vi "Main.vi"(8 "error in (no error)":errorcluster, 11 "ExampleClassC in":refnum<class "ExampleClassC.lvclass">) -> (0 "error out":errorcluster, 3 "component":refnum<class "ExampleClassC.lvclass">)   [LabVIEW 2012, in "ExampleClassC.lvclass"]
doc: "Main VI of the component. This should contain the GUI of your component and be called when creating an executable."
uses:
  ExampleClassC.lvclass
  <vilib>/Distrio/Murmex/InitialiseMessage/InitialiseMessage.lvclass
  ExampleClassC.lvclass/ExampleClassC.ctl
  <vilib>/Distrio/Murmex/TerminateMessage/TerminateMessage.lvclass
  <vilib>/Distrio/Murmex/ConfigureMessage/ConfigureMessage.lvclass
  <vilib>/Distrio/Murmex/StopMessage/StopMessage.lvclass
  <vilib>/Distrio/Murmex/StartMessage/StartMessage.lvclass
  <vilib>/Distrio/Murmex/Murmex/Set log reference.vi
  <vilib>/Distrio/Murmex/Murmex/Set VI reference.vi
  <vilib>/Distrio/Murmex/Murmex/Set configure at initialise.vi
  <vilib>/Distrio/Murmex/Murmex/Set relay start stop to observers.vi
  <vilib>/Distrio/Murmex/Murmex/Murmex.lvclass
  <vilib>/Distrio/Murmex/Message/Message.lvclass
panel:
  in  "button:configure":bool
  in  "button:start":bool
  in  "image":path
  in  "button:quit":bool
  in  "terminate?":bool
  in  "ID":string
  out "log":string
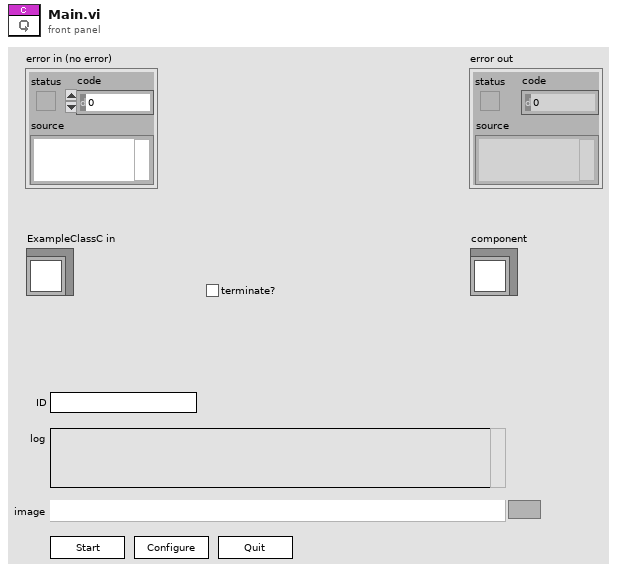
[diagram p1: front panel]
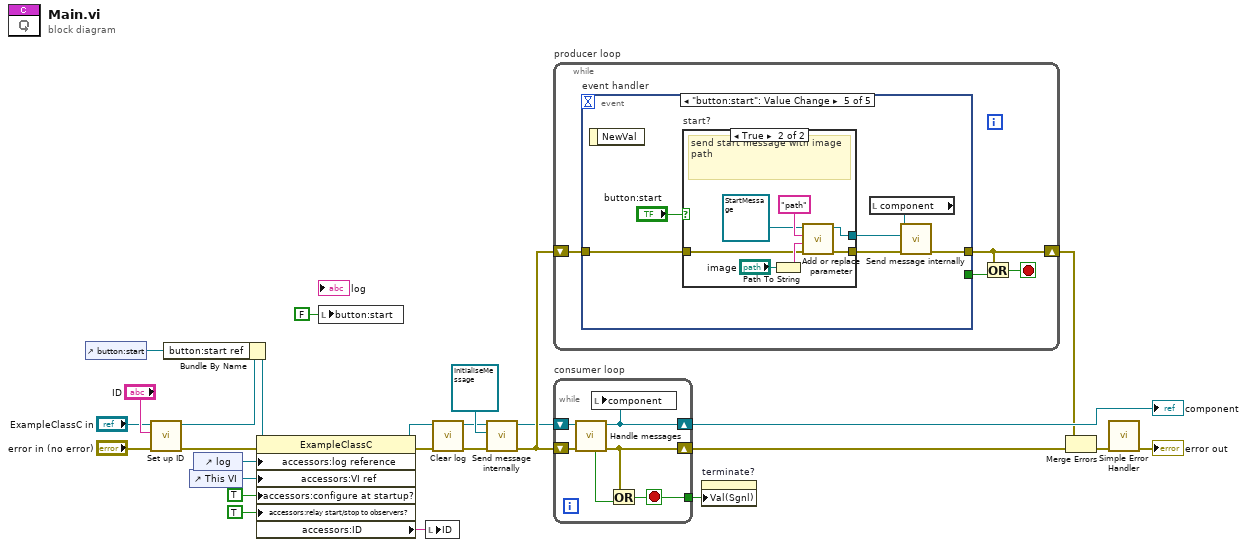
[diagram p0: block diagram]
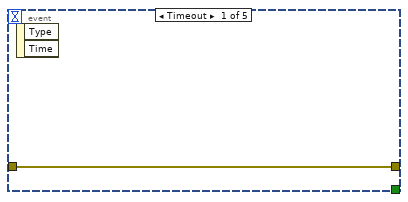
[diagram p2: hidden frame]
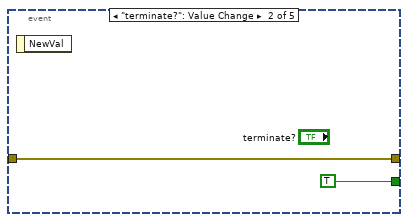
[diagram p3: hidden frame]
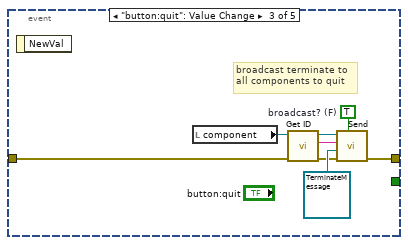
[diagram p4: hidden frame]
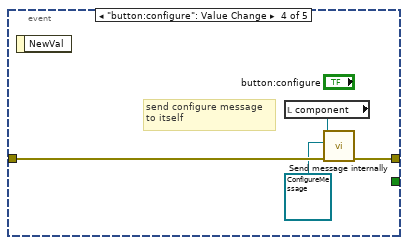
[diagram p5: hidden frame]
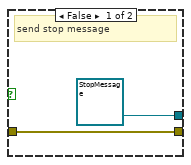
[diagram p6: hidden frame]
diagram:
  n1 = control-ref of="button:start"() -> (w4:refnum<vi>)
  n2 = call <vilib>:"Set up ID.vi"("error in (no error)"="error in (no error)", "component ID"="ID", "MurmexBase in"="ExampleClassC in") -> ("error out"=w22:errorcluster, "MurmexBase out"=w6:refnum<class "ExampleClassC.lvclass">)  [unwired: 6 in, 1 out]
  n3 = Bundle By Name(cluster=w6, "button:start ref"=w4) -> (w5:refnum<class "ExampleClassC.lvclass">)
  n4 = control-ref of="This VI"() -> (w24:refnum<vi>)
  n5 = control-ref of="log"() -> (w25:refnum<vi>)
  n6 = property class="ExampleClassC"(reference=w5, error in=w22, "accessors:log reference"=w25, "accessors:VI ref"=w24, "accessors:configure at startup?"=TRUE ("configure at startup?"), "accessors:relay start/stop to observers?"=TRUE ("relay start/stop to observers?")) -> (reference out=w13:refnum<class "ExampleClassC.lvclass">, error out=w19:errorcluster, "accessors:ID"=w20:string)
  n7 = local write "button:start"(FALSE ("button:start")) -> ()
  n8 = local write "ID"(w20) -> ()
  n9 = call <vilib>:"Clear log.vi"("error in (no error)"=w19, "MurmexBase in"=w13) -> ("error out"=w14:errorcluster, "MurmexBase out"=w12:refnum<class "ExampleClassC.lvclass">)  [unwired: 8 in]
  n10 = call <vilib>:"Send message internally.vi"("error in (no error)"=w14, "Message"=refnum<class "InitialiseMessage.lvclass"> refnum ("Distrio Murmex 1.5:InitialiseMessage"), "Murmex in"=w12) -> ("error out"=w17:errorcluster, "Murmex out"=w16:refnum<class "ExampleClassC.lvclass">)  [unwired: 7 in]
  n11 = while "producer loop" {
    shift-right: [w29] -> w3
    shift-left: w17 -> [w30]
    stop <- w27 stop-if-true
    n12 = event "event handler" shown="[4] \"button:start\": Value Change" {
      selector: _ -> [_ _ _ _ _]
      dyn-events: _ -> [_ _ _ _ _]
      timeout: _ -> [_ _ _ _ _]
      tunnel: [w31 w33 w40 w44 w48] -> w29
      tunnel: w30 -> [w31 w33 w41 w45 w51]
      tunnel: [_ TRUE _ _ _] -> w28
      event Timeout {
        n13 = event-data() -> ()  [unwired: 1 in, 2 out]
      }
      event "terminate?": Value Change {
        n14 = event-data() -> ()  [unwired: 1 in, 1 out]
      }
      event "button:quit": Value Change {
        w35 = TRUE  # broadcast? (F)
        # "broadcast terminate to\nall components to quit"
        n15 = event-data() -> ()  [unwired: 1 in, 1 out]
        n16 = local read "component"() -> (w34:refnum<class "ExampleClassC.lvclass">)
        n17 = call <vilib>:"Get ID.vi"("error in (no error)"=w41, "Murmex in"=w34) -> ("error out"=w38:errorcluster, "component id"=w36:string, "Murmex out"=w37:refnum<class "ExampleClassC.lvclass">)  [unwired: 7 in]
        n18 = call <vilib>:"Send.vi"("broadcast? (F)"=w35, "error in (no error)"=w38, "Message"=refnum<class "TerminateMessage.lvclass"> refnum ("Distrio Murmex 1.5:TerminateMessage"), "recipient"=w36, "Murmex in"=w37) -> ("error out"=w40:errorcluster)  [unwired: 5 in, 1 out]
      }
      event "button:configure": Value Change {
        # "send configure message\nto itself"
        n19 = event-data() -> ()  [unwired: 1 in, 1 out]
        n20 = local read "component"() -> (w42:refnum<class "ExampleClassC.lvclass">)
        n21 = call <vilib>:"Send message internally.vi"("error in (no error)"=w45, "Message"=refnum<class "ConfigureMessage.lvclass"> refnum ("Distrio Murmex 1.5:ConfigureMessage"), "Murmex in"=w42) -> ("error out"=w44:errorcluster)  [unwired: 7 in, 1 out]
      }
      event "button:start": Value Change {
        n22 = event-data() -> ()  [unwired: 1 in, 1 out]
        n23 = case "start?" shown="True" "button:start" {
          tunnel: w51 -> [w53 w55]
          tunnel: [w53 w60] -> w49
          tunnel: [refnum<class "StopMessage.lvclass"> refnum ("Distrio Murmex 1.5:StopMessage") w56] -> w47
          frame False {
            # "send stop message"
          }
          frame True {
            # "send start message with image path"
            n24 = Path To String(path="image") -> (string=w57:string)
            n25 = call <vilib>:"Add or replace parameter.vi"("error in (no error)"=w55, "value"=w57, "name"="path", "Message in"=refnum<class "StartMessage.lvclass"> refnum ("Distrio Murmex 1.5:StartMessage")) -> ("error out"=w60:errorcluster, "Message out"=w56:refnum<class "StartMessage.lvclass">)  [unwired: 6 in]
          }
        }
        n26 = local read "component"() -> (w46:refnum<class "ExampleClassC.lvclass">)
        n27 = call <vilib>:"Send message internally.vi"("error in (no error)"=w49, "Message"=w47, "Murmex in"=w46) -> ("error out"=w48:errorcluster)  [unwired: 7 in, 1 out]
      }
    }
    n28 = Or(x=w29, y=w28) -> (x .or. y?=w27:bool)
  }
  n29 = while "consumer loop" {
    shift-right: [w64] -> w2
    shift-left: w17 -> [w66]
    shift-right: [w61] -> w26
    shift-left: w16 -> [w65]
    tunnel: [w62] -> w18
    stop <- w62 stop-if-true
    n30 = call <vilib>:"Handle messages.vi"("error in (no error)"=w66, "Murmex in"=w65) -> ("error out"=w64:errorcluster, "Murmex out"=w61:refnum<class "ExampleClassC.lvclass">, "terminated?"=w63:bool)  [unwired: 7 in]
    n31 = local write "component"(w61) -> ()
    n32 = Or(x=w64, y=w63) -> (x .or. y?=w62:bool)
  }
  "component" <- w26
  n33 = property on="terminate?" class="Bool (strict)"("Val(Sgnl)"=w18) -> ()  [unwired: 2 in, 2 out]
  n34 = Merge Errors(w3, w2) -> (w1:errorcluster)
  n35 = call <vilib>:"Simple Error Handler.vi"("error in (no error)"=w1) -> ("error out"=→"error out":errorcluster)  [unwired: 4 in, 4 out]
